vi "Apply CFR to Waveform.vi"(0 "Waveform In":T2={"Waveform Name"="Wfm", "Waveform"={"x0"=0.0, "dx"=0.0, "y"=[]}, "Signal Bandwidth (Hz)"=0.0, "PAPR (dB)"=0.0, "Burst Length (s)"=0.0, "Sample Rate"=0.0, "Burst Start Locations"=[], "Burst Stop Locations"=[], "Idle Duration Present?"=FALSE} {"Sample Rate" format="%#_6p"; "Burst Length (s)" format="%#_6p"; "PAPR (dB)" format="%.2f"; "Signal Bandwidth (Hz)" format="%.2f"; "Waveform"."y" format="%.2f"; "Waveform"."dx" format="%^.2e"; "Waveform"."x0" format="%^.2e"}, 5 "Pre-DPD CFR":T1={"CFR Enabled"=0, "CFR Method"=0, "Max Iterations"=10, "Target PAPR (dB)"=8.0, "Peak Windowing"={"Window Type"=7, "Window Length"=10}, "Sigmoid"={"Shaping Factor"=5.0, "Shaping Threshold (dB)"=-5.0}, "Filter Enabled"=0, "Signal Settings"={"Carrier"=[{"Carrier Offset (Hz)"=0.0, "Carrier Bandwidth (Hz)"=20000000.0}], "Number of Carriers"=1.0}} {"Signal Settings"."Carrier"."Carrier Bandwidth (Hz)" format="%.2p"; "Signal Settings"."Carrier"."Carrier Offset (Hz)" format="%.2p"; "Filter Enabled" items=["False", "True"]; "Peak Windowing"."Window Type" items=["Flat Top"=1, "Hanning"=2, "Hamming"=3, "Gaussian"=4, "Blackman"=5, "Blackman-Harris"=6, "Kaiser-Bessel"=7]; "CFR Method" items=["Clipping", "Peak Windowing", "Sigmoid"]; "CFR Enabled" items=["False", "True"]}, 11 "error in (no error)":errorcluster) -> (4 "Waveform Out":T2={"Waveform Name"="Wfm", "Waveform"={"x0"=0.0, "dx"=0.0, "y"=[]}, "Signal Bandwidth (Hz)"=0.0, "PAPR (dB)"=0.0, "Burst Length (s)"=0.0, "Sample Rate"=0.0, "Burst Start Locations"=[], "Burst Stop Locations"=[], "Idle Duration Present?"=FALSE} {"Sample Rate" format="%#_6p"; "Burst Length (s)" format="%#_6p"; "PAPR (dB)" format="%.2f"; "Signal Bandwidth (Hz)" format="%.2f"; "Waveform"."y" format="%.2f"; "Waveform"."dx" format="%^.2e"; "Waveform"."x0" format="%^.2e"}, 15 "error out":errorcluster)   [LabVIEW 2018, in "SG.lvlib"]
uses:
  SG.lvlib
  Typedefs/Waveform.ctl
  Typedefs/Pre DPD CFR Configuration.ctl
  <vilib>/RFmx/SpecAn/mx/RFmxSpecAn.llb/RFmxSpecAn Select Measurement (Single).vi
  <resource>/objmgr/RFmxSpecAn.rc
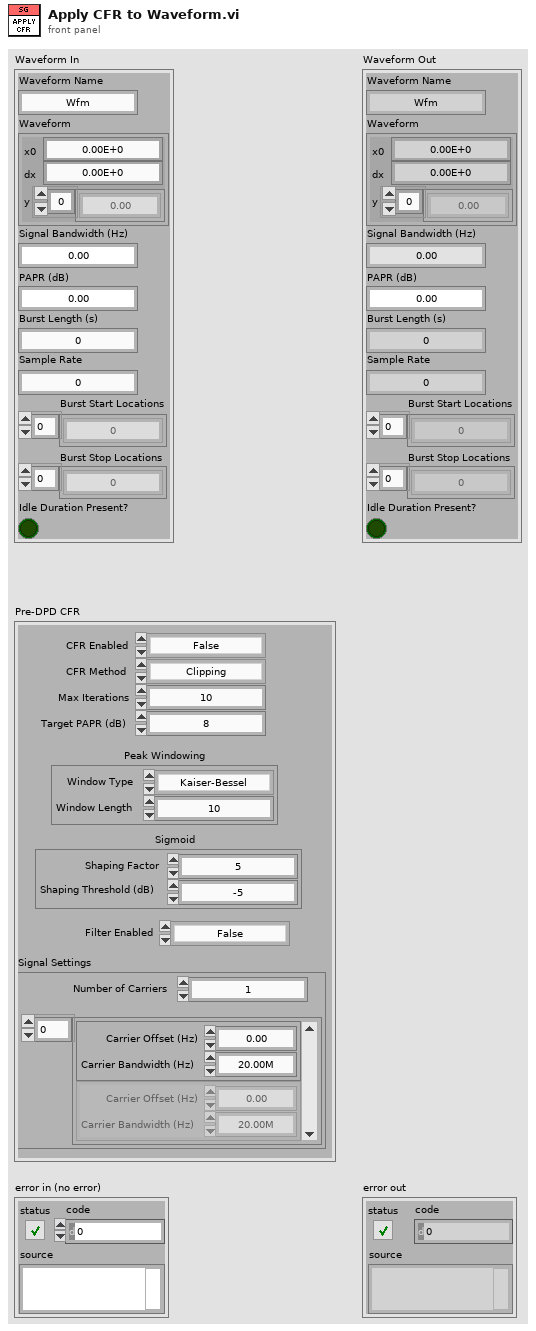
[diagram p1: front panel]
types:
  T1 = typedef "SG.lvlib/Pre DPD CFR Configuration.ctl" = cluster{"CFR Enabled":i32, "CFR Method":i32, "Max Iterations":i32, "Target PAPR (dB)":dbl, "Peak Windowing":cluster{"Window Type":i32, "Window Length":i32}, "Sigmoid":cluster{"Shaping Factor":dbl, "Shaping Threshold (dB)":dbl}, "Filter Enabled":i32, "Signal Settings":cluster{"Carrier":cluster{"Carrier Offset (Hz)":dbl, "Carrier Bandwidth (Hz)":dbl}[], "Number of Carriers":dbl}}
  T2 = typedef "SG.lvlib/Waveform.ctl" = cluster{"Waveform Name":string, "Waveform":cluster{"x0":dbl, "dx":dbl, "y":csg[]}, "Signal Bandwidth (Hz)":dbl, "PAPR (dB)":dbl, "Burst Length (s)":dbl, "Sample Rate":dbl, "Burst Start Locations":i32[], "Burst Stop Locations":i32[], "Idle Duration Present?":bool}
  T3 = enum16{"ACP", "CCDF", "CHP", "FCnt", "Harmonics", "OBW", "SEM", "Spectrum", "Spur", "TXP", "AMPM", "DPD", "IQ", "IM", "NF", "PhaseNoise"}
  T4 = cluster{"Carrier Offset (Hz)":dbl, "Carrier Bandwidth (Hz)":dbl}[]
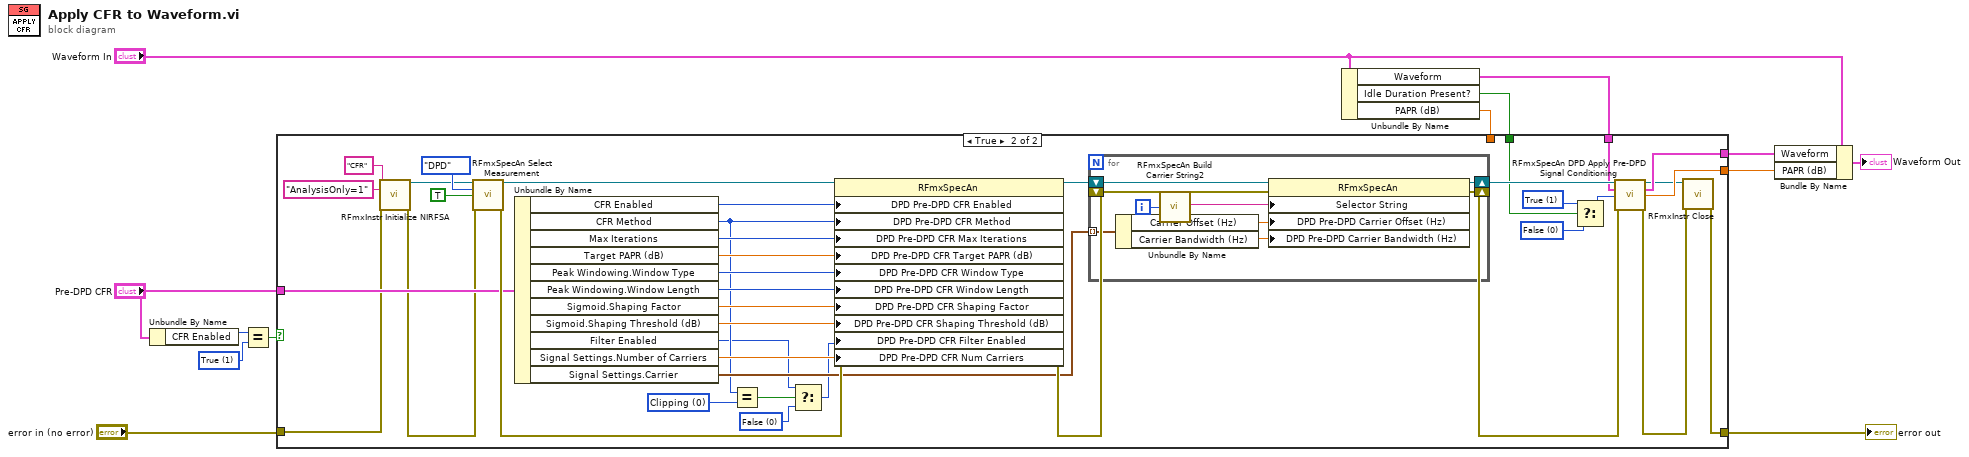
[diagram p0: block diagram]
diagram:
  w11 = 1 items=["False", "True"] ("CFR Enabled")
  n1 = Unbundle By Name("Pre-DPD CFR") -> ("CFR Enabled"=w13:i32)
  n2 = Equal?(x=w13, y=w11) -> (x = y?=w12:bool)
  n3 = Unbundle By Name("Waveform In") -> ("Waveform"=w8:cluster{"x0":dbl, "dx":dbl, "y":csg[]}, "Idle Duration Present?"=w7:bool, "PAPR (dB)"=w1:dbl)
  n4 = case shown="True" w12 {
    tunnel: [w15 w27] -> w6
    tunnel: "error in (no error)" -> [w15 w22]
    tunnel: [w16 w39] -> w3
    tunnel: [w14 w38] -> w2
    tunnel: "Pre-DPD CFR" -> [_ w37]
    tunnel: w8 -> [w16 w21]
    tunnel: w7 -> [_ w18]
    tunnel: w1 -> [w14 _]
    frame False {
    }
    frame True {
      w19 = 1 items=["False", "True"] ("Idle Duration Present")
      w17 = 0 items=["False", "True"] ("Idle Duration Present")
      w31 = 0 items=["False", "True"] ("DPD Pre-DPD CFR Filter Enabled")
      w34 = 0 items=["Clipping", "Peak Windowing", "Sigmoid"] ("DPD Pre-DPD CFR Method")
      n5 = call <vilib>:"RFmxInstr Initialize NIRFSA.vi"("Resource Name"="CFR" ("Option String"), "Option String"="AnalysisOnly=1", "error in (no error)"=w22) -> ("Instrument Handle Out"=w26:refnum<k21>, "error out"=w23:errorcluster)  [unwired: 10 in, 1 out]
      n6 = call-poly <vilib>:"RFmxSpecAn Select Measurement.vi"("Instrument Handle In"=w26, "Measurement"=T3."DPD", "Enable All Traces"=TRUE, "error in (no error)"=w23) -> ("Instrument Handle Out"=w53:refnum<k21>, "error out"=w52:errorcluster)  [unwired: 10 in]
      n7 = Unbundle By Name(w37) -> ("CFR Enabled"=w47:i32, "CFR Method"=w35:i32, "Max Iterations"=w46:i32, "Target PAPR (dB)"=w45:dbl, "Peak Windowing.Window Type"=w44:i32, "Peak Windowing.Window Length"=w43:i32, "Sigmoid.Shaping Factor"=w42:dbl, "Sigmoid.Shaping Threshold (dB)"=w41:dbl, "Filter Enabled"=w32:i32, "Signal Settings.Number of Carriers"=w40:dbl, "Signal Settings.Carrier"=w36:T4)
      n8 = Equal?(x=w35, y=w34) -> (x = y?=w33:bool)
      n9 = Select(t=w32, s=w33, f=w31) -> (s? t:f=w30:i32)
      n10 = property class="RFmxSpecAn"(reference=w53, error in=w52, "DPD Pre-DPD CFR Enabled"=w47, "DPD Pre-DPD CFR Method"=w35, "DPD Pre-DPD CFR Max Iterations"=w46, "DPD Pre-DPD CFR Target PAPR (dB)"=w45, "DPD Pre-DPD CFR Window Type"=w44, "DPD Pre-DPD CFR Window Length"=w43, "DPD Pre-DPD CFR Shaping Factor"=w42, "DPD Pre-DPD CFR Shaping Threshold (dB)"=w41, "DPD Pre-DPD CFR Filter Enabled"=w30, "DPD Pre-DPD CFR Num Carriers"=w40) -> (reference out=w49:refnum<k21>, error out=w51:errorcluster)
      n11 = for {
        shift-right: [w63] -> w50
        shift-left: w51 -> [w64]
        shift-right: [w61] -> w48
        shift-left: w49 -> [w62]
        tunnel: w36 -> [w58] mode=indexing
        i -> [w60]
        n12 = Unbundle By Name(w58) -> ("Carrier Offset (Hz)"=w57:dbl, "Carrier Bandwidth (Hz)"=w56:dbl)
        n13 = call <vilib>:"RFmxSpecAn Build Carrier String2.vi"("Carrier Number"=w60) -> ("Selector String Out"=w59:string)  [unwired: 14 in]
        n14 = property class="RFmxSpecAn"(reference=w62, error in=w64, "Selector String"=w59, "DPD Pre-DPD Carrier Offset (Hz)"=w57, "DPD Pre-DPD Carrier Bandwidth (Hz)"=w56) -> (reference out=w61:refnum<k21>, error out=w63:errorcluster)
      }
      n15 = Select(t=w19, s=w18, f=w17) -> (s? t:f=w20:i32)
      n16 = call <vilib>:"RFmxSpecAn DPD Apply Pre-DPD Signal Conditioning.vi"("Instrument Handle In"=w48, "Waveform In"=w21, "Idle Duration Present"=w20, "error in (no error)"=w50) -> ("Instrument Handle Out"=w29:refnum<k21>, "Waveform Out"=w39:cluster{"x0":dbl, "dx":dbl, "y":csg[]}, "PAPR (dB)"=w38:dbl, "error out"=w28:errorcluster)  [unwired: 8 in]
      n17 = call <vilib>:"RFmxInstr Close.vi"("Instrument Handle In"=w29, "error in (no error)"=w28) -> ("error out"=w27:errorcluster)  [unwired: 13 in]
    }
  }
  "error out" <- w6
  n18 = Bundle By Name(cluster="Waveform In", "Waveform"=w3, "PAPR (dB)"=w2) -> (→"Waveform Out":T2)
